vi "ImageCollect16Stream2008.vi"() -> ()   [LabVIEW 2009]
doc: "The HL Sequence VI acquires multiple images and displays them in an array of image controls. A sequence is appropriate for applications where you must perform processing on multiple images. You can configure a sequence to acquire every frame or to skip a variable number of frames between each image.\n\nIMAQ Create creates multiple image buffers. The array of image buffers is wired to IMAQ Sequence. The Skip Table input to IMAQ Sequence specifies the number of frames to skip between captures. IMAQ Sequence acquires and returns the images. An image control displays the array of images on the front panel. IMAQ Sequence performs a synchronous acquisition. To acquire asynchronously, refer to the LL Sequence VI in the IMAQ Low Level.llb."
panel:
  out "Fractional Change 2":dbl[][](graph)
  out "Saving":bool
  out "Fractional Change 4":dbl[][](graph)
  out "Fractional Change 3":dbl[][](graph)
  in  "DATA Path 2":path=path "E:/Capture/test.avi"
  out "Rep Number":dbl
  out "Running":bool
  out "Bin Size, Frames":i32=29
  in  "Which Bin":i32=2
  out "Fractional Change 1":dbl[][](graph)
  in  "Raw Bin#":i32
  out "Displays Averaged":dbl[][](graph)
  in  "Secs to record":u16=10 min=1 max=600
  in  "Trigger action":u32(ring)=1 items=["Disabled", "Trigger start of acquisition", "Trigger start of each buffer list", "Trigger each buffer", "Trigger each line (linescan)", "Trigger end of acquisition"]
  in  "Trigger Type":u32(ring) items=["External", "RTSI", "ISO In"]
  in  "stop":bool
  in  "Interface Name":string="img0"
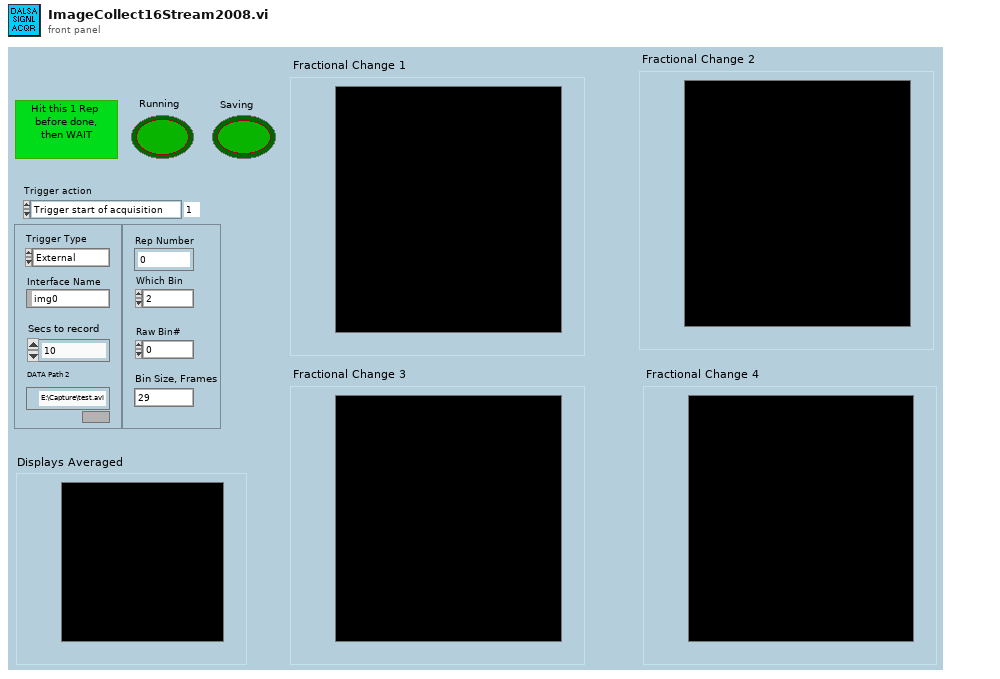
[diagram p1: front panel]
types:
  T1 = enum16{"big-endian, network order", "native, host order", "little-endian"}
  T2 = typedef "IMAQ Image.ctl" = refnum<image>
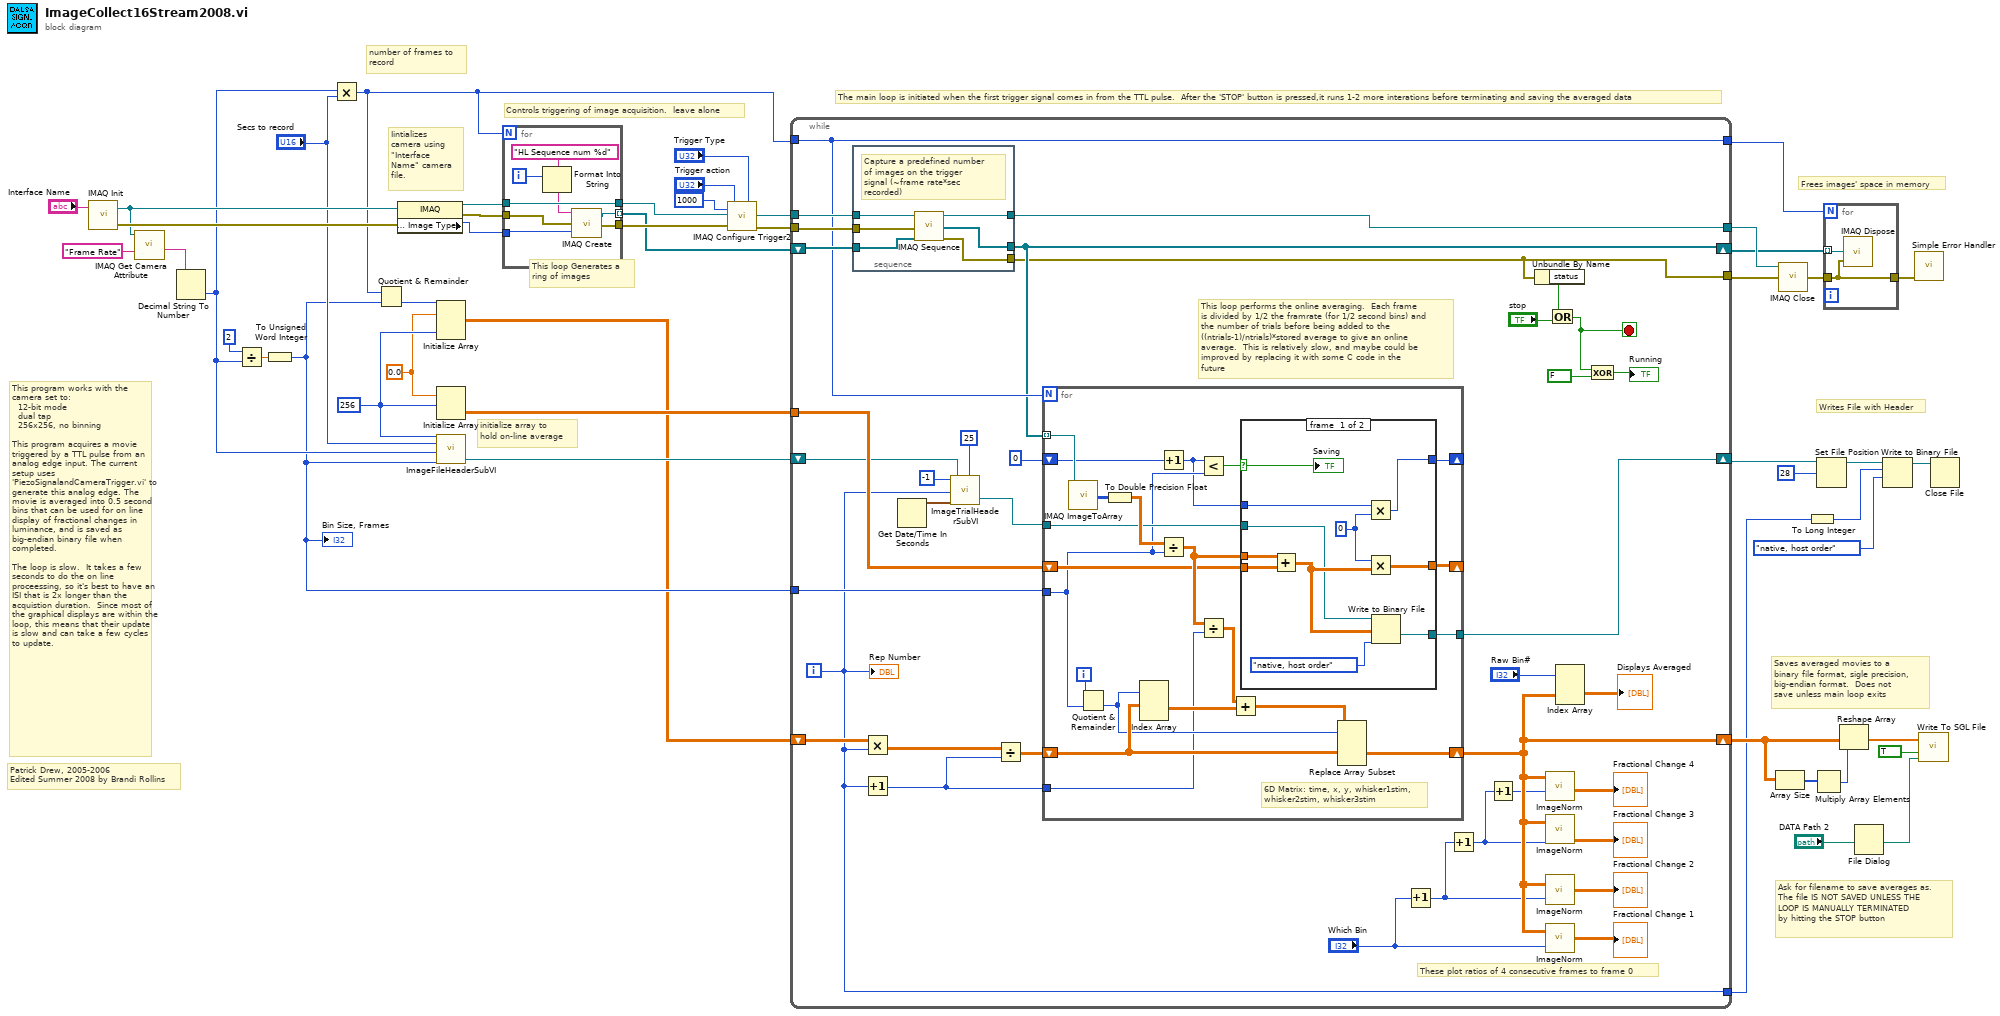
[diagram p0: block diagram]
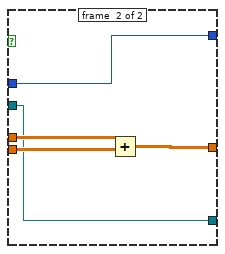
[diagram p2: hidden frame]
diagram:
  w8 = 256 ("dimension size")
  w7 = 0.0 ("element")
  # "number of frames to record"
  # "Writes File with Header"
  # "This loop Generates a ring of images"
  # "Frees images' space in memory"
  # "Patrick Drew, 2005-2006\nEdited Summer 2008 by Brandi Rollins"
  # "Controls triggering of image acquisition.  leave alone"
  # "This program works with the camera set to: \n  12-bit mode \n  dual tap\n  256x256, no binning\n\nThis program acquires a movie triggered by a TTL pulse from an analog edge input. The current setup uses 'PiezoSignalandCameraTrigger.vi' to generate this analog edge. The movie is averaged into 0.5 second  bins that can be used for on line display of fractional changes in luminance, and is saved as big-endian binary file when completed. \n\nThe loop is slow.  It takes a few seconds to do the on line proceessing, so it's best to have an ISI that is 2x longer than the acquistion duration.  Since most of the graphical displays are within the loop, this means that their update is slow and can take a few cycles to update."
  # "Saves averaged movies to a binary file format, sigle precision, big-endian format.  Does not save unless main loop exits"
  # "The main loop is initiated when the first trigger signal comes in from the TTL pulse.  After the 'STOP' button is pressed,it runs 1-2 more interations before terminating and saving the averaged data"
  # "Ask for filename to save averages as.\nThe file IS NOT SAVED UNLESS THE LOOP IS MANUALLY TERMINATED\nby hitting the STOP button"
  # "initialize array to hold on-line average"
  # "Iintializes camera using \"Interface Name\" camera file."
  n1 = call <vilib>:"IMAQ Init.vi"("Interface Name"="Interface Name") -> ("error out"=w18:errorcluster, "IMAQ Session Out"=w17:refnum<k11>)  [unwired: 9 in]
  n2 = call <vilib>:"IMAQ Get Camera Attribute.vi"("Camera Attribute"="Frame Rate", "IMAQ Session In"=w17) -> ("Attribute Value"=w1:string)  [unwired: 5 in, 2 out]
  n3 = Decimal String To Number(string=w1) -> (number=w13:i32)  [unwired: 2 in, 1 out]
  n4 = Divide(x=w13, y=2) -> (x/y=w36:dbl)
  n5 = To Unsigned Word Integer(number=w36) -> (unsigned 16bit integer=w3:u16)
  "Bin Size, Frames" <- w3
  n6 = Multiply(x=w13, y="Secs to record") -> (x*y=w16:i32)
  n7 = Quotient & Remainder(x=w16, y=w3) -> (floor(x/y)=w38:i32)  [unwired: 1 out]
  n8 = property class="IMAQ"(reference=w17, error in=w18) -> (reference out=w46:refnum<k11>, error out=w47:errorcluster, "Image Parameters : Image Type"=w28:u32)
  n9 = Initialize Array(w7, w38, w8, w8) -> (w2:dbl[][][])
  n10 = Initialize Array(w7, w8, w8) -> (w15:dbl[][])
  n11 = call "ImageFileHeaderSubVI.vi"("size x"=w8, "size y"=w8, "frame rate"=w13, "bin duration"=w3, "recording duration"="Secs to record") -> ("refnum out"=w27:refnum<file>)  [unwired: 2 in]
  n12 = for {
    N: w16 -> [_]
    tunnel: [w56] -> w14
    tunnel: [w55] -> w10 mode=indexing
    tunnel: w47 -> [w54]
    tunnel: w46 -> [w53]
    tunnel: [w53] -> w6
    tunnel: w28 -> [w52]
    i -> [w51]
    n13 = Format Into String(format string="HL Sequence num %d", w51) -> (resulting string=w49:string)  [unwired: 2 in, 1 out]
    n14 = call "IMAQ Create"("Image Name"=w49, "Image Type"=w52, "error in (no error)"=w54) -> ("New Image"=w55:T2, "error out"=w56:errorcluster)  [unwired: 2 in]
  }
  n15 = call <vilib>:"IMAQ Configure Trigger2.vi"("Frame timeout (ms)"=u32 1000, "Trigger action"="Trigger action", "error in (no error)"=w14, "Trigger Type"="Trigger Type", "IMAQ Session In"=w6) -> ("error out"=w12:errorcluster, "IMAQ Session Out"=w43:refnum<k11>)  [unwired: 5 in]
  n16 = while {
    tunnel: w43 -> [w80]
    tunnel: w12 -> [w81]
    tunnel: w16 -> [w64]
    shift-right: [w67] -> w31
    shift-left: w2 -> [w92]
    shift-right: [w62] -> w9
    shift-left: w10 -> [w93]
    tunnel: w3 -> [w88]
    tunnel: [w63] -> w40
    tunnel: [w60] -> w11
    tunnel: [w64] -> w4
    tunnel: w15 -> [w75]
    shift-right: [w68] -> w26
    shift-left: w27 -> [w71]
    tunnel: [w59] -> w21
    i -> [w59]
    stop <- w85 stop-if-true
    # "This loop performs the online averaging.  Each frame is divided by 1/2 the framrate (for 1/2 second bins) and the number of trials before being added to the ((ntrials-1)/ntrials)*stored average to give an online average.  This is relatively slow, and maybe could be improved by replacing it with some C code in the future"
    # "These plot ratios of 4 consecutive frames to frame 0"
    n17 = stacked-sequence {
      tunnel: w80 -> [w136]
      tunnel: w81 -> [w135]
      tunnel: [w134] -> w60
      tunnel: [w133] -> w62
      tunnel: w93 -> [w132]
      tunnel: [w131] -> w63
      frame #0 {
        # "Capture a predefined number of images on the trigger signal (~frame rate*sec recorded)"
        n18 = call <vilib>:"IMAQ Sequence.vi"("error in (no error)"=w135, "Images In"=w132, "IMAQ Session In"=w136) -> ("error out"=w134:errorcluster, "Images Out"=w133:T2[], "IMAQ Session Out"=w131:refnum<k11>)  [unwired: 6 in]
      }
    }
    n19 = Multiply(x=w92, y=w59) -> (x*y=w91:dbl[][][])
    n20 = Increment(x=w59) -> (x+1=w89:i32)
    n21 = Get Date/Time In Seconds() -> (seconds since 1Jan1904=w69:timestamp)
    n22 = call "ImageTrialHeaderSubVI.vi"("Bytes to skip"=i64 25 ("offset (in bytes) (0)"), "Time Stamp"=w69, "stim number"=-1, "trial"=w59, "refnum in"=w71) -> ("refnum out"=w72:refnum<file>)
    n23 = Divide(x=w91, y=w89) -> (x/y=w90:dbl[][][])
    n24 = for {
      N: w64 -> [_]
      tunnel: w62 -> [w114] mode=indexing
      tunnel: w89 -> [w107]
      shift-right: [w110] -> w67
      shift-left: w90 -> [w112]
      tunnel: w88 -> [w97]
      shift-right: [w100] -> _
      shift-left: w75 -> [w101]
      shift-right: [w94] -> _
      shift-left: 0 -> [w96]
      tunnel: w72 -> [w99]
      tunnel: [w98] -> w68
      i -> [w103]
      # "6D Matrix: time, x, y, whisker1stim,\nwhisker2stim, whisker3stim"
      n25 = call "IMAQ ImageToArray"("Image"=w114) -> ("Image Pixels (I16)"=w106:i16[][])  [unwired: 3 in, 4 out]
      n26 = Quotient & Remainder(x=w103, y=w97) -> (floor(x/y)=w111:i32)  [unwired: 1 out]
      n27 = To Double Precision Float(number=w106) -> (double precision float=w105:dbl[][])
      n28 = Index Array(array=w112, index (dim 0)=w111) -> (element=w113:dbl[][])  [unwired: 2 in]
      n29 = Increment(x=w96) -> (x+1=w95:i32)
      n30 = Divide(x=w105, y=w97) -> (x/y=w102:dbl[][])
      n31 = Less?(x=w95, y=w97) -> (x < y?=w104:bool)
      n32 = Divide(x=w102, y=w107) -> (x/y=w108:dbl[][])
      n33 = Add(x=w108, y=w113) -> (x+y=w109:dbl[][])
      n34 = case shown="False" w104 {
        selector: w104 -> [w115 _]
        tunnel: w102 -> [w122 w130]
        tunnel: w101 -> [w123 w129]
        tunnel: [w120 w128] -> w100
        tunnel: w95 -> [w125 w127]
        tunnel: [w124 w127] -> w94
        tunnel: w99 -> [w117 w126]
        tunnel: [w116 w126] -> w98
        frame #0 {
          w121 = 0 ("y")
          n35 = Add(x=w123, y=w122) -> (x+y=w119:dbl[][])
          n36 = Multiply(x=w125, y=w121) -> (x*y=w124:i32)
          n37 = Multiply(x=w121, y=w119) -> (x*y=w120:dbl[][])
          n38 = Write to Binary File(file (use dialog)=w117, data=w119, 9:T1."native, host order" ("byte order (0:big-endian, network order)")) -> (refnum out=w116:refnum<file>)  [unwired: 3 in, 2 out]
          "Saving" <- w115
        }
        frame #1 {
          n39 = Add(x=w129, y=w130) -> (x+y=w128:dbl[][])
        }
      }
      n40 = Replace Array Subset(array=w112, new element=w109, index (dim 0)=w111) -> (w110:dbl[][][])  [unwired: 2 in]
    }
    n41 = Increment(x="Which Bin") -> (x+1=w66:i32)
    n42 = Increment(x=w66) -> (x+1=w58:i32)
    n43 = Increment(x=w58) -> (x+1=w57:i32)
    n44 = Unbundle By Name(w60) -> ("status"=w82:bool)
    n45 = call "ImageNorm.vi"("Numeric"=w57, "Array"=w67) -> ("Fractional Change 2"=→"Fractional Change 4":dbl[][])
    n46 = call "ImageNorm.vi"("Numeric"=w58, "Array"=w67) -> ("Fractional Change 2"=→"Fractional Change 3":dbl[][])
    n47 = call "ImageNorm.vi"("Numeric"=w66, "Array"=w67) -> ("Fractional Change 2"=→"Fractional Change 2":dbl[][])
    n48 = call "ImageNorm.vi"("Numeric"="Which Bin", "Array"=w67) -> ("Fractional Change 2"=→"Fractional Change 1":dbl[][])
    n49 = Or(x=w82, y="stop") -> (x .or. y?=w85:bool)
    n50 = Index Array(array=w67, index (dim 0)="Raw Bin#") -> (element=→"Displays Averaged":dbl[][])  [unwired: 2 in]
    n51 = Exclusive Or(1:FALSE, 2:w85) -> (0:→"Running":bool)
    "Rep Number" <- w59
  }
  n52 = Array Size(array=w31) -> (size(s)=w29:i32[])
  n53 = call <vilib>:"IMAQ Close.vi"("error in (no error)"=w11, "IMAQ Session In"=w40) -> ("error out"=w45:errorcluster)  [unwired: 9 in]
  n54 = To Long Integer(number=w21) -> (32bit integer=w20:i32)
  n55 = Multiply Array Elements(1:w29) -> (0:w34:i32)
  n56 = Set File Position(offset (in bytes) (0)=i64 28, refnum=w26) -> (refnum out=w24:refnum<file>)  [unwired: 2 in, 1 out]
  n57 = for {
    N: w4 -> [_]
    tunnel: w45 -> [w138]
    tunnel: [w138] -> w44
    tunnel: w9 -> [w137] mode=indexing
    n58 = call "IMAQ Dispose"("Image"=w137, "error in (no error)"=w138) -> ()  [unwired: 4 in, 1 out]
  }
  n59 = Reshape Array(w31, w34) -> (w30:dbl[])
  n60 = File Dialog(11:"DATA Path 2") -> (3:w32:path)  [unwired: 6 in, 3 out]
  n61 = Write to Binary File(file (use dialog)=w24, data=w20, 9:T1."native, host order" ("byte order (0:big-endian, network order)")) -> (refnum out=w23:refnum<file>)  [unwired: 3 in, 2 out]
  n62 = call <vilib>:"Simple Error Handler.vi"("error in (no error)"=w44) -> ()  [unwired: 4 in, 5 out]
  n63 = call <vilib>:"Write To SGL File.vi"("append to file? (new file:F)"=TRUE, "1D array"=w30, "file path (dialog if empty)"=w32) -> ()  [unwired: 4 in, 1 out]
  n64 = Close File(refnum=w23) -> ()  [unwired: 1 in, 2 out]
